vi "Check if Position in Range.vi"(9 "Dir(Fwd=T)":bool, 10 "Target Position":i32, 11 "Cur Encoder Value":i32) -> (2 "Soft Limit?":bool, 3 "In Range?":bool)   [LabVIEW 2015, in "Tool Module.lvlib"]
uses:
  Tool Module.lvlib
  Support/ToolModGLOB.vi
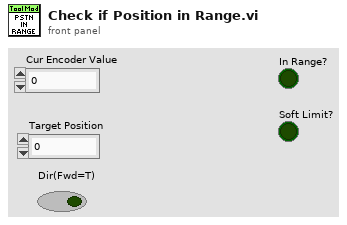
[diagram p1: front panel]
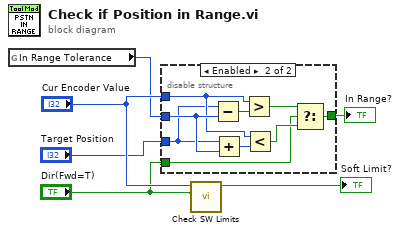
[diagram p0: block diagram]
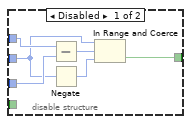
[diagram p2: hidden frame]
diagram:
  n1 = global read "ToolModGLOB.vi" "In Range Tolerance"() -> (w2:i32)
  n2 = disable-structure shown="Enabled" {
    disable-tunnel: [w12 w17] -> w6
    disable-tunnel: "Cur Encoder Value" -> [w9 w15]
    disable-tunnel: "Target Position" -> [w8 w14]
    disable-tunnel: w2 -> [w7 w16]
    disable-tunnel: "Dir(Fwd=T)" -> [_ w13]
    frame Disabled {
      n3 = Subtract(x=w9, y=w8) -> (x-y=w10:i32)
      n4 = Negate(x=w7) -> (-x=w11:i32)
      n5 = In Range and Coerce(upper limit=w7, x=w10, lower limit=w11) -> (In Range?=w12:bool)  [unwired: 1 out]
    }
    frame Enabled {
      n6 = Subtract(x=w14, y=w16) -> (x-y=w19:i32)
      n7 = Add(x=w14, y=w16) -> (x+y=w18:i32)
      n8 = Greater?(x=w15, y=w19) -> (0:w20:bool)
      n9 = Less?(x=w15, y=w18) -> (x < y?=w21:bool)
      n10 = Select(t=w20, s=w13, f=w21) -> (s? t:f=w17:bool)
    }
  }
  "In Range?" <- w6
  n11 = call "Check SW Limits.vi"("Dir(Fwd=T)"="Dir(Fwd=T)", "Encoder in"="Cur Encoder Value") -> ("Soft Limit?"=→"Soft Limit?":bool)  [unwired: 9 in]
